vi "transformCoords_3d.vi"(8 "transform properties":T1={"theta (deg)"=0.0, "X sc factor (px/step)"=1.0, "Y sc factor (px/step)"=1.0, "zero loc (x,y,z)"=[0.0, 0.0], "flip y?"=FALSE, "flip x?"=FALSE, "gamma (deg)"=25.0, "flip z?"=FALSE, "Z sc factor (px/step)"=0.1098, "actuator"={"Actuator COM"="COM3", "Actuator type"=enum."Scientifica"}, "safe space (steps)"=[-69533, 0, -29190]} {"Y sc factor (px/step)" format="%#_13g"; "X sc factor (px/step)" format="%#_13g"; "theta (deg)" format="%#_13g"}, 9 "z":i32, 10 "y":i32, 11 "x":i32) -> (1 "z out":dbl, 2 "y out":dbl, 3 "x out":dbl)   [LabVIEW 2015]
uses:
  <vilib>/Analysis/NI_AALPro.lvlib
  <vilib>/Analysis/coordinate.llb/2D Cartesian Coordinate Rotation (Scalar).vi
  pipette cleaning/pressure box/cleaning_soft/controls/actuator_type.ctl
  pipette cleaning/pressure box/cleaning_soft/controls/actuator_cluster.ctl
  transform_properties_actuators.ctl
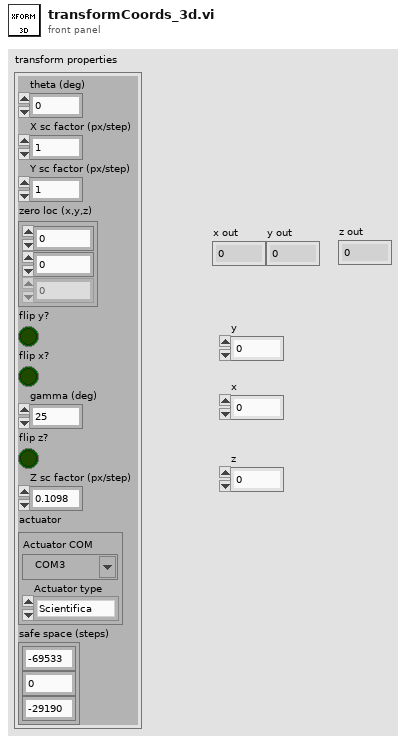
[diagram p1: front panel]
types:
  T1 = typedef "transform_properties_actuators.ctl" = cluster{"theta (deg)":dbl, "X sc factor (px/step)":dbl, "Y sc factor (px/step)":dbl, "zero loc (x,y,z)":dbl[], "flip y?":bool, "flip x?":bool, "gamma (deg)":dbl, "flip z?":bool, "Z sc factor (px/step)":dbl, "actuator":T2, "safe space (steps)":i32[]}
  T2 = typedef "actuator_cluster.ctl" = cluster{"Actuator COM":refnum<visa-resource-name>, "Actuator type":T3}
  T3 = typedef "actuator_type.ctl" = enum16{"Scientifica", "Sutter", "Demo", "Off"}
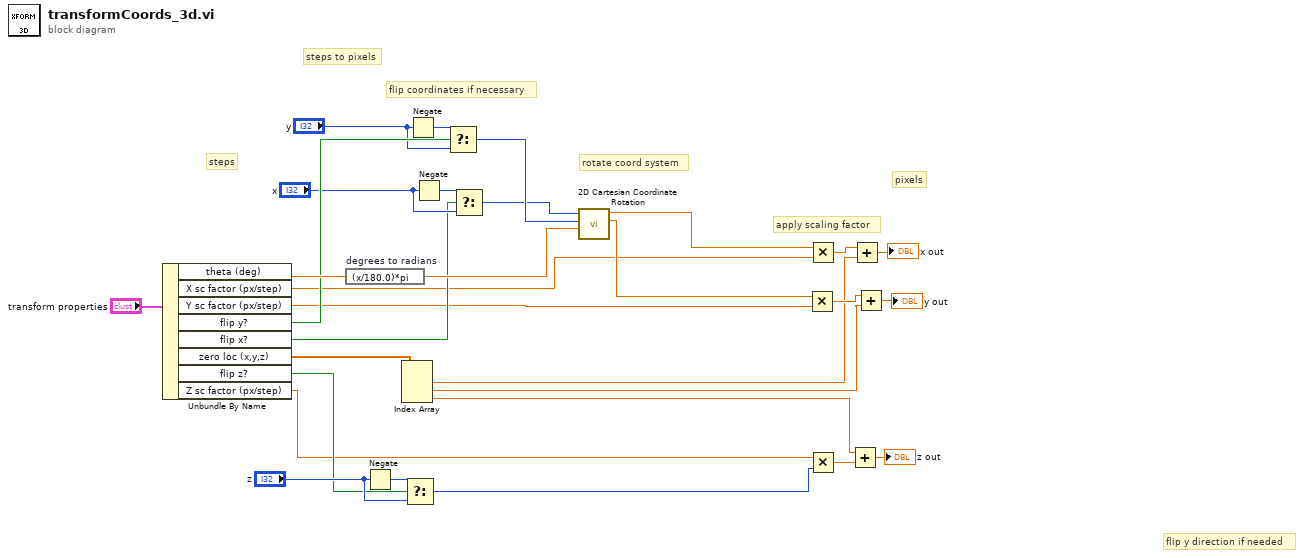
[diagram p0: block diagram]
diagram:
  # "steps"
  # "pixels"
  # "steps to pixels"
  # "flip coordinates if necessary"
  # "flip y direction if needed"
  # "apply scaling factor"
  # "rotate coord system"
  n1 = Unbundle By Name("transform properties") -> ("theta (deg)"=w26:dbl, "X sc factor (px/step)"=w10:dbl, "Y sc factor (px/step)"=w9:dbl, "flip y?"=w24:bool, "flip x?"=w18:bool, "zero loc (x,y,z)"=w13:dbl[], "flip z?"=w5:bool, "Z sc factor (px/step)"=w1:dbl)
  n2 = expression code="(x/180.0)*pi" "degrees to radians"(w26) -> (w29:dbl)
  n3 = Negate(x="z") -> (-x=w7:i32)
  n4 = Index Array(array=w13) -> (element #1=w12:dbl, element #2=w11:dbl, element #3=w4:dbl)  [unwired: 3 in]
  n5 = Select(t=w7, s=w5, f="z") -> (s? t:f=w2:i32)
  n6 = Negate(x="y") -> (-x=w25:i32)
  n7 = Negate(x="x") -> (-x=w21:i32)
  n8 = Select(t=w25, s=w24, f="y") -> (s? t:f=w22:i32)
  n9 = Select(t=w21, s=w18, f="x") -> (s? t:f=w19:i32)
  n10 = call-poly <vilib>:"2D Cartesian Coordinate Rotation.vi"("theta"=w29, "y"=w22, "x"=w19) -> ("y out"=w27:dbl, "x out"=w28:dbl)  [unwired: 6 in, 1 out]
  n11 = Multiply(x=w27, y=w9) -> (x*y=w15:dbl)
  n12 = Multiply(x=w28, y=w10) -> (x*y=w17:dbl)
  n13 = Multiply(x=w1, y=w2) -> (x*y=w3:dbl)
  n14 = Add(x=w4, y=w3) -> (x+y=→"z out":dbl)
  n15 = Add(x=w17, y=w12) -> (x+y=→"x out":dbl)
  n16 = Add(x=w15, y=w11) -> (x+y=→"y out":dbl)
